vi "_Raise Dom Content Loaded.vi"(4 "Events":T1, 5 "Event Data":cluster{"sender":refnum<k24>, "e":refnum<k24>}, 6 "Control Ref":refnum<k24>, 7 "Event Common Data":T2) -> ()   [LabVIEW 2020, in "WebView2 Control.xctl"]
uses:
  WebView2 Control.xctl
  E:/Labview/LV 2020/Libs/WebView2/LV-WebView2/Source/Libs/Microsoft.Web.WebView2.Core.dll
  Libs/Microsoft.Web.WebView2.Core.dll
  Events.ctl
  Navigation Event Data.ctl
  Source Changed Event Data.ctl
  Navigation Start Event Data.ctl
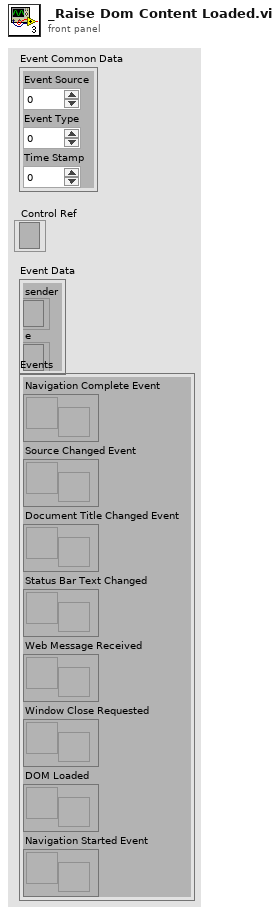
[diagram p1: front panel]
types:
  T1 = typedef "WebView2 Control.xctl/Events.ctl" = cluster{"Navigation Complete Event":refnum<user-event>, "Source Changed Event":refnum<user-event>, "Document Title Changed Event":refnum<user-event>, "Status Bar Text Changed":refnum<user-event>, "Web Message Received":refnum<user-event>, "Window Close Requested":refnum<user-event>, "DOM Loaded":refnum<user-event>, "Navigation Started Event":refnum<user-event>}
  T2 = cluster{"Event Source":i32, "Event Type":u32, "Time Stamp":u32}
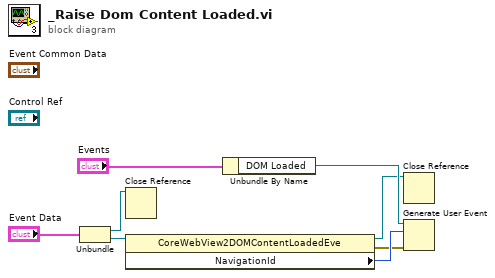
[diagram p0: block diagram]
diagram:
  n1 = Unbundle("Event Data") -> ("sender"=w4:refnum<k24>, "e"=w5:refnum<k24>)
  n2 = Close Reference(reference=w4) -> ()  [unwired: 1 in, 1 out]
  n3 = property class="CoreWebView2DOMContentLoadedEve"(reference=w5) -> (reference out=w3:refnum<k24>, error out=w1:errorcluster, "NavigationId"=w2:u64)  [unwired: 1 in]
  n4 = Unbundle By Name("Events") -> ("DOM Loaded"=w7:refnum<user-event>)
  n5 = Close Reference(reference=w3) -> ()  [unwired: 1 in, 1 out]
  n6 = Generate User Event(user event=w7, event data cluster=w2, error in=w1) -> ()  [unwired: 1 in, 2 out]
